vi "override timing.vi"(6 "Priority":u64, 8 "error in (no error)":errorcluster, 9 "Offset":u64, 10 "Decimation":u64=1, 11 "Mock Plugin in":refnum<class "Mock Plugin.lvclass">) -> (0 "error out":errorcluster, 3 "Mock Plugin out":refnum<class "Mock Plugin.lvclass">)   [LabVIEW 2017, in "Mock Plugin.lvclass"]
uses:
  Plugin/Mock Plugin.lvclass
  Classes/Plugin/Plugin.lvclass
  Classes/Timing/Timing.lvclass
  C:/Git/DSF/Data Sharing Framework Core/Classes/Plugin/Plugin.lvclass
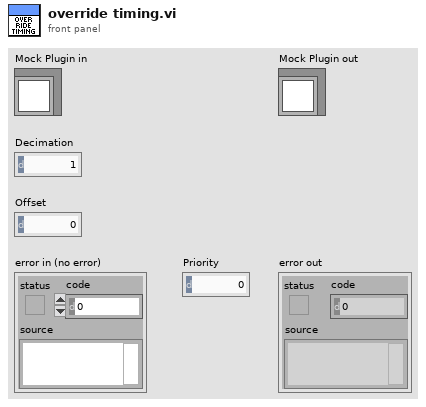
[diagram p1: front panel]
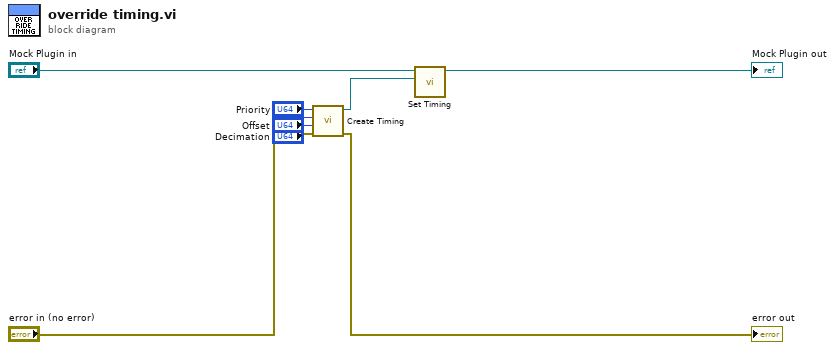
[diagram p0: block diagram]
diagram:
  n1 = call "Create Timing.vi"("error in (no error)"="error in (no error)", "offset"="Offset", "decimation"="Decimation", "Timing in"="Priority") -> ("error out"=→"error out":errorcluster, "Timing out"=w5:refnum<class "Timing.lvclass">)  [unwired: 6 in]
  n2 = call "Set Timing.vi"("Timing"=w5, "Plugin in"="Mock Plugin in") -> ("Plugin out"=→"Mock Plugin out":refnum<class "Mock Plugin.lvclass">)  [unwired: 9 in]
